vi "UnittodB(1DDBL).vi"(11 "Data(U)":dbl[](array[numeric])) -> (3 "Data(dBU)":dbl[](array[numeric]))   [LabVIEW 2015]
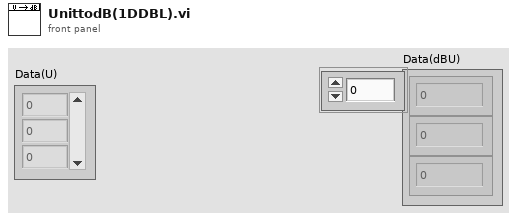
[diagram p1: front panel]
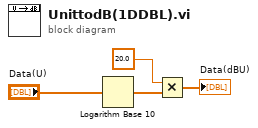
[diagram p0: block diagram]
diagram:
  n1 = Logarithm Base 10(1:"Data(U)") -> (0:w2:dbl[])
  n2 = Multiply(x=20.0, y=w2) -> (x*y=→"Data(dBU)":dbl[])
